vi "Resize Columns.vi"(6 "Default Option":T1, 8 "Error In":errorcluster, 10 "Data":variant, 11 "State In":T2) -> (0 "Error Out":errorcluster, 3 "State Out":T2)   [LabVIEW 2018, in "Bookmark Manager.lvlib"]
uses:
  Bookmark Manager.lvlib
  Controls/State.ctl
  <vilib>/addons/analyzer/_analyzerctrls.llb/VIAnCtl Analysis App Info.ctl
  Controls/Bookmark.ctl
  Controls/VI Identifier.ctl
  Controls/Bookmarks Groups.ctl
  Controls/Column Resizing Options.ctl
  <vilib>/Utility/miscctls.llb/LVRectTypeDef.ctl
  Preferences Keys.vi
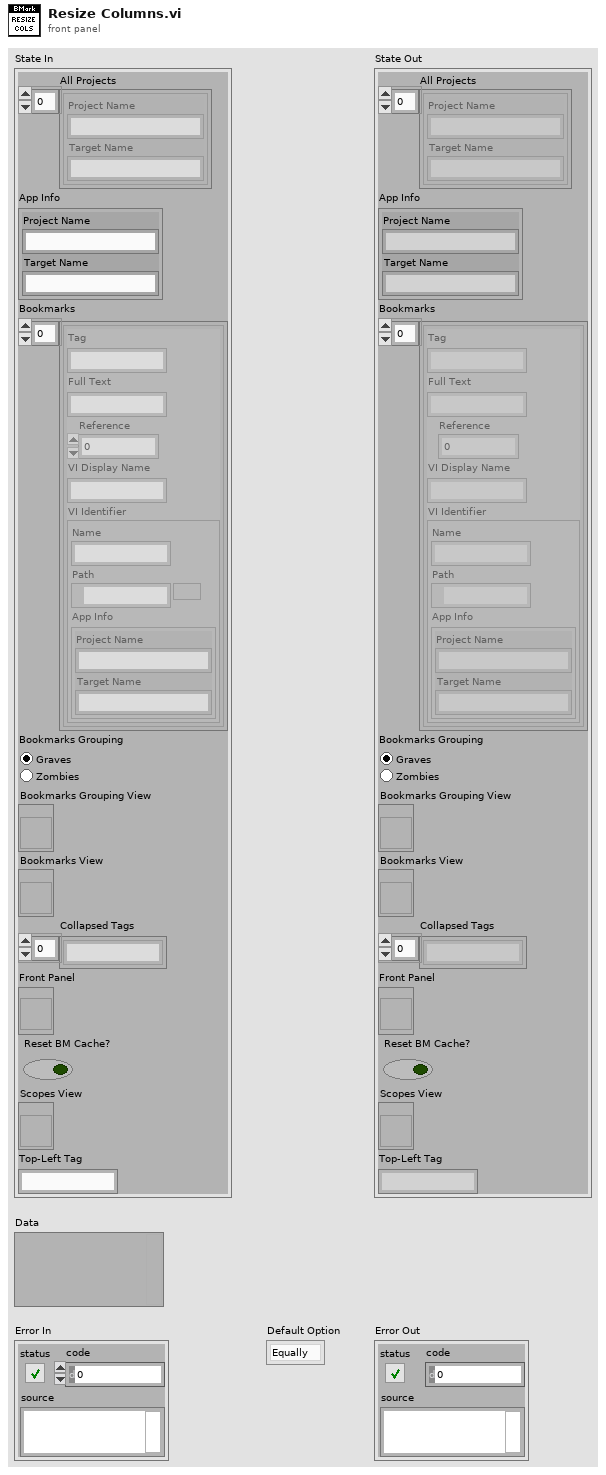
[diagram p1: front panel]
types:
  T1 = typedef "Bookmark Manager.lvlib/Column Resizing Options.ctl" = enum16{"Equally", "Last"}
  T2 = typedef "Bookmark Manager.lvlib/State.ctl" = cluster{"All Projects":T3[], "App Info":T3, "Bookmarks":T4[], "Bookmarks Grouping":T6, "Bookmarks Grouping View":refnum<vi>, "Bookmarks View":refnum<vi>, "Collapsed Tags":string[], "Front Panel":refnum<vi>, "Reset BM Cache?":bool, "Scopes View":refnum<vi>, "Top-Left Tag":string}
  T3 = typedef "VIAnCtl Analysis App Info.ctl" = cluster{"Project Name":string, "Target Name":string}
  T4 = typedef "Bookmark Manager.lvlib/Bookmark.ctl" = cluster{"Tag":string, "Full Text":string, "Reference":i32, "VI Display Name":string, "VI Identifier":T5}
  T5 = typedef "Bookmark Manager.lvlib/VI Identifier.ctl" = cluster{"Name":string, "Path":path, "App Info":T3}
  T6 = typedef "Bookmark Manager.lvlib/Bookmarks Groups.ctl" = enum32{"Graves", "Zombies"}
  T7 = typedef "LVRectTypeDef.ctl" = cluster{"Left":i16, "Top":i16, "Right":i16, "Bottom":i16}
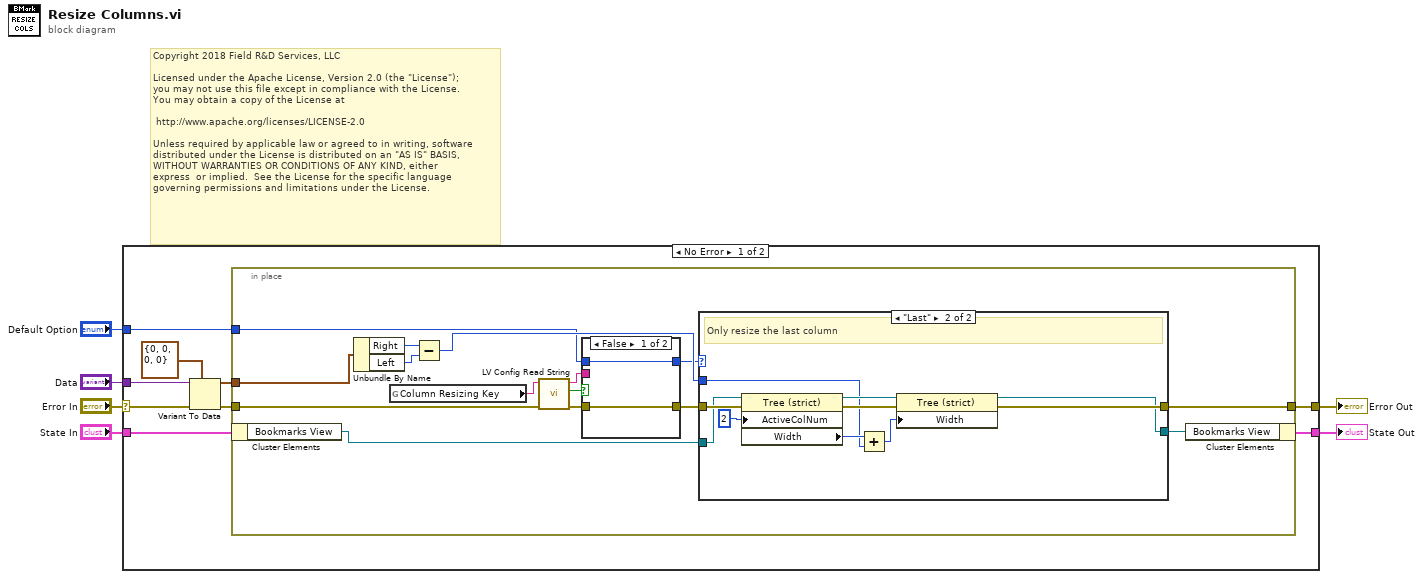
[diagram p0: block diagram]
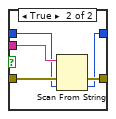
[diagram p2: hidden frame]
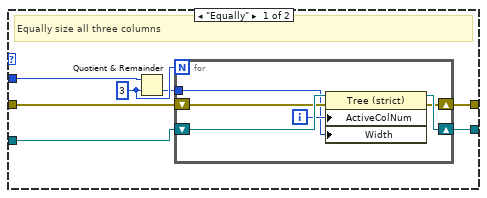
[diagram p3: hidden frame]
diagram:
  # "Copyright 2018 Field R&D Services, LLC\n\nLicensed under the Apache License, Version 2.0 (the \"License\");\nyou may not use this file except in compliance with the License.\nYou may obtain a copy of the License at\n\n\thttp://www.apache.org/licenses/LICENSE-2.0\n\nUnless required by applicable law or agreed to in writing, software\ndistributed under the License is distributed on an \"AS IS\" BASIS,\nWITHOUT WARRANTIES OR CONDITIONS OF ANY KIND, either \nexpress  or implied.  See the License for the specific language \ngoverning permissions and limitations under the License."
  n1 = case shown="No Error" "Error In" {
    selector: "Error In" -> [w8 w61]
    tunnel: [w15 w61] -> w6
    tunnel: "Data" -> [w12 _]
    tunnel: [w10 w62] -> w4
    tunnel: "State In" -> [w9 w62]
    tunnel: "Default Option" -> [w7 _]
    frame No Error {
      n2 = Variant To Data(error in=w8, type=T7 {"Left"=0, "Top"=0, "Right"=0, "Bottom"=0} ("NewBnds"), Variant=w12) -> (data=w13:T7, error out=w14:errorcluster)
      n3 = in-place {
        in-place-border: w13 -> [w25]
        in-place-border: w14 -> [w23]
        in-place-border: [w24] -> w15
        in-place-border: w7 -> [w17]
        n4 = in-place-cluster #1(w9) -> ("Bookmarks View"=w27:refnum<vi>)
        n5 = Unbundle By Name(w25) -> ("Right"=w30:i16, "Left"=w29:i16)
        n6 = global read "Preferences Keys.vi" "Column Resizing Key"() -> (w21:string)
        n7 = Subtract(x=w30, y=w29) -> (x-y=w28:i16)
        n8 = call <resource>:"LV Config Read String.vi"("error in"=w23, "key"=w21) -> ("error out"=w22:errorcluster, "found?"=w16:bool, "value"=w19:string)  [unwired: 3 in]
        n9 = case shown="False" w16 {
          tunnel: w22 -> [w32 w37]
          tunnel: [w32 w36] -> w20
          tunnel: w19 -> [_ w35]
          tunnel: [w31 w34] -> w18
          tunnel: w17 -> [w31 w33]
          frame False {
          }
          frame True {
            n10 = Scan From String(input string=w35, error in=w37, default 1=w33) -> (error out=w36:errorcluster, output 1=w34:T1)  [unwired: 2 in, 2 out]
          }
        }
        n11 = case shown="\"Last\"" w18 {
          tunnel: w28 -> [w44 w51]
          tunnel: w27 -> [w43 w52]
          tunnel: [w42 w53] -> w26
          tunnel: w20 -> [w41 w55]
          tunnel: [w40 w54] -> w24
          frame "Equally" {
            w39 = i16 3 ("y")
            # "Equally size all three columns"
            n12 = Quotient & Remainder(x=w44, y=w39) -> (floor(x/y)=w38:i16)  [unwired: 1 out]
            n13 = for {
              N: w39 -> [_]
              shift-right: [w49] -> w42
              shift-left: w43 -> [w50]
              shift-right: [w47] -> w40
              shift-left: w41 -> [w48]
              tunnel: w38 -> [w45]
              i -> [w46]
              n14 = property class="Tree (strict)"(reference=w50, error in=w48, "ActiveColNum"=w46, "Width"=w45) -> (reference out=w49:refnum<vi>, error out=w47:errorcluster)
            }
          }
          frame "Last" {
            # "Only resize the last column"
            n15 = property class="Tree (strict)"(reference=w52, error in=w55, "ActiveColNum"=2 ("Active Cell:Active Column Number")) -> (reference out=w58:refnum<vi>, error out=w60:errorcluster, "Width"=w57:i32)
            n16 = Add(x=w57, y=w51) -> (x+y=w59:i32)
            n17 = property class="Tree (strict)"(reference=w58, error in=w60, "Width"=w59) -> (reference out=w53:refnum<vi>, error out=w54:errorcluster)
          }
        }
        n18 = in-place-cluster #1("Bookmarks View"=w26) -> (w10:T2)
      }
    }
    frame Error {
    }
  }
  "Error Out" <- w6
  "State Out" <- w4
